vi "取最小值.vi"(2 "距离":dbl[](array[numeric]), 3 "角度":dbl[](array[numeric])) -> (0 "最小值角度":dbl, 1 "最小值距离":dbl)   [LabVIEW 2016]
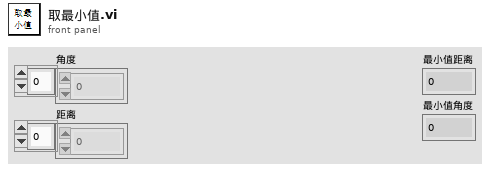
[diagram p1: front panel]
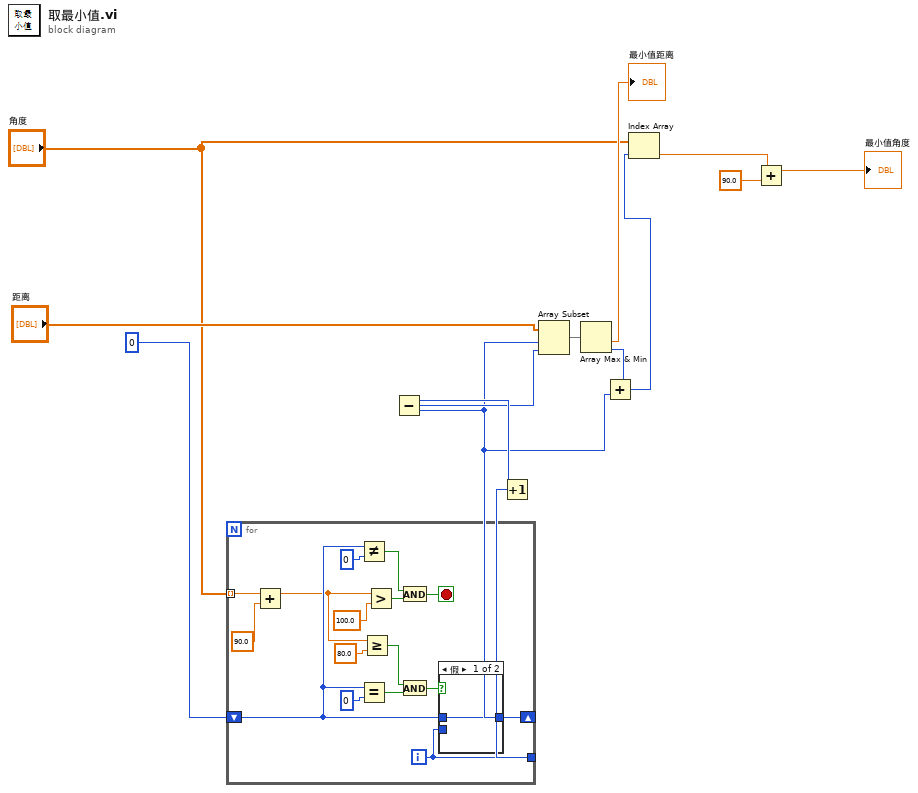
[diagram p0: block diagram]
diagram:
  n1 = for {
    tunnel: "角度" -> [w21] mode=indexing
    shift-right: [w25] -> w5
    shift-left: 0 -> [w17]
    tunnel: [w18] -> w13
    i -> [w18]
    stop <- w19 stop-if-true
    n2 = Add(x=w21, y=90.0) -> (x+y=w16:dbl)
    n3 = Not Equal?(x=w17, y=0) -> (x != y?=w23:bool)
    n4 = Equal?(x=w17, y=0) -> (x = y?=w27:bool)
    n5 = Greater Or Equal?(x=w16, y=80.0) -> (x >= y?=w29:bool)
    n6 = Greater?(x=w16, y=100.0) -> (0:w22:bool)
    n7 = And(x=w23, y=w22) -> (x .and. y?=w19:bool)
    n8 = And(x=w29, y=w27) -> (x .and. y?=w26:bool)
    n9 = case shown="假" w26 {
      tunnel: w18 -> [_ w32]
      tunnel: [w31 w32] -> w25
      tunnel: w17 -> [w31 _]
      frame False {
      }
      frame True {
      }
    }
  }
  n10 = Increment(x=w13) -> (x+1=w11:i32)
  n11 = Subtract(x=w11, y=w5) -> (x-y=w10:i32)
  n12 = Array Subset(array="距离", index=w5, length=w10) -> (w9:dbl[])
  n13 = Array Max & Min(array=w9) -> (min value=→"最小值距离":dbl, min index (indices)=w4:i32)  [unwired: 2 out]
  n14 = Add(x=w4, y=w5) -> (x+y=w3:i32)
  n15 = Index Array(array="角度", index=w3) -> (element=w6:dbl)
  n16 = Add(x=w6, y=90.0) -> (x+y=→"最小值角度":dbl)
